vi "Measurement Logic.vi"() -> ()   [LabVIEW 2020, in "VISA Measurement.lvlib"]
uses:
  VISA Measurement.lvlib
  Measurement Configuration.ctl
  Measurement Results.ctl
  <vilib>/MeasurementLink/MeasurementLink Measurement Server/Measure Call Context/Measure Call Context.lvclass
  <vilib>/MeasurementLink/MeasurementLink VISA/Initialize Sessions - 1Sess.vi
  <vilib>/Instr/_visa.llb/VISA Configure Serial Port (Instr).vi
  <vilib>/MeasurementLink/MeasurementLink VISA/MeasurementLink VISA.lvlib
  <vilib>/MeasurementLink/MeasurementLink Session Management V1/Session Reservation/Session Reservation.lvclass
panel:
  out "measure call context out":refnum<class "Measure Call Context.lvclass">
  in  "measure call context in":refnum<class "Measure Call Context.lvclass">
  out "measurement results":T1
  in  "measurement configuration":T2={"pin name"="", "command"="*IDN?", "baud rate"=9600, "data bits"=8, "parity"=enum."None", "stop bits"=0, "flow control"=0, "read byte count"=1000, "end read on term char"=TRUE, "end write on term char"=TRUE} {"flow control" items=["None", "XON/XOFF", "RTS/CTS", "XON/XOFF & RTS/CTS", "DTR/DSR", "XON/XOFF & DTR/DSR"]; "stop bits" items=["1.0"=10, "1.5"=15, "2.0"=20]}
  out "error out":errorcluster
  in  "error in":errorcluster
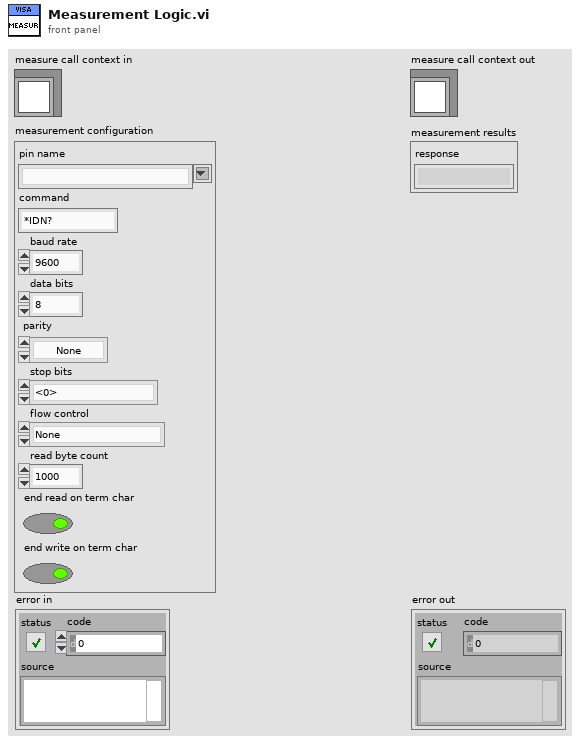
[diagram p1: front panel]
types:
  T1 = typedef "VISA Measurement.lvlib/Measurement Results.ctl" = cluster{"response":string}
  T2 = typedef "VISA Measurement.lvlib/Measurement Configuration.ctl" = cluster{"pin name":string, "command":string, "baud rate":u32, "data bits":u32, "parity":enum32{"None", "Odd", "Even", "Mark", "Space"}, "stop bits":u32, "flow control":u32, "read byte count":u32, "end read on term char":bool, "end write on term char":bool}
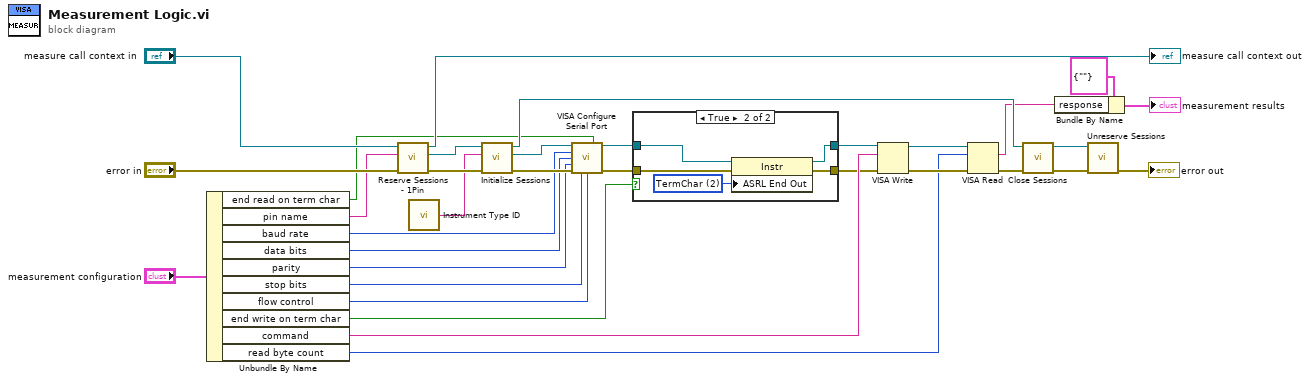
[diagram p0: block diagram]
diagram:
  n1 = Unbundle By Name("measurement configuration") -> ("end read on term char"=w2:bool, "pin name"=w21:string, "baud rate"=w20:u32, "data bits"=w19:u32, "parity"=w18:enum32{"None", "Odd", "Even", "Mark", "Space"}, "stop bits"=w17:u32, "flow control"=w16:u32, "end write on term char"=w3:bool, "command"=w15:string, "read byte count"=w4:u32)
  n2 = call <vilib>:"Reserve Sessions - 1Pin.vi"("error in"="error in", "pin or relay name"=w21, "measurement context in"="measure call context in") -> ("error out"=w31:errorcluster, "session reservation out"=w32:refnum<class "Session Reservation.lvclass">, "measurement context out"=→"measure call context out":refnum<class "Measure Call Context.lvclass">)  [unwired: 6 in]
  n3 = call "Instrument Type ID.vi"() -> ("instrument type id"=w1:string)  [unwired: 5 in]
  n4 = call-poly <vilib>:"Initialize Sessions.vi"("error in"=w31, "instrument type id"=w1, "session reservation in"=w32) -> ("error out"=w29:errorcluster, "session"=w30:refnum<visa-resource-name>, "session reservation out"=w23:refnum<class "Session Reservation.lvclass">)  [unwired: 5 in, 1 out]
  n5 = call-poly "VISA Configure Serial Port"("VISA resource name"=w30, "Enable Termination\nChar (T)"=w2, "baud rate (9600)"=w20, "data bits (8)"=w19, "parity (0:none)"=w18, "error in (no error)"=w29, "stop bits (10: 1 bit)"=w17, "flow control (0:none)"=w16) -> ("VISA resource name out"=w8:refnum<visa-resource-name>, "error out"=w7:errorcluster)  [unwired: 1 in, 5 out]
  n6 = case shown="True" w3 {
    tunnel: w8 -> [w35 w40]
    tunnel: w7 -> [w34 w39]
    tunnel: [w35 w38] -> w6
    tunnel: [w34 w37] -> w5
    frame False {
    }
    frame True {
      w36 = u16 2 items=["None", "Last Bit", "TermChar", "Break"] ("Serial Settings:End Mode for Writes")
      n7 = property class="Instr"(reference=w40, error in=w39, "ASRL End Out"=w36) -> (reference out=w38:refnum<visa-resource-name>, error out=w37:errorcluster)
    }
  }
  n8 = VISA Write(VISA resource name=w6, write buffer=w15, error in (no error)=w5) -> (VISA resource name out=w10:refnum<visa-resource-name>, error out=w9:errorcluster)  [unwired: 1 out]
  n9 = VISA Read(VISA resource name=w10, byte count=w4, error in (no error)=w9) -> (read buffer=w12:string, error out=w28:errorcluster)  [unwired: 2 out]
  n10 = call <vilib>:"Close Sessions.vi"("error in"=w28, "session reservation in"=w23) -> ("error out"=w27:errorcluster, "session reservation out"=w26:refnum<class "Session Reservation.lvclass">)  [unwired: 8 in]
  n11 = Bundle By Name(cluster=T1 {"response"=""} ("Measurement Results"), "response"=w12) -> (→"measurement results":T1)
  n12 = call <vilib>:"Unreserve Sessions.vi"("error in"=w27, "session reservation in"=w26) -> ("error out"=→"error out":errorcluster)  [unwired: 9 in]
